vi "Update.vi"(8 "error in (no error)":errorcluster caption="entrée d'erreur (pas d'erreur)", 11 "Dual Fan en entrée":refnum<class "Dual Fan.lvclass">) -> (0 "error out":errorcluster caption="sortie d'erreur", 3 "Dual Fan en sortie":refnum<class "Dual Fan.lvclass">)   [LabVIEW 2015, in "Dual Fan.lvlib" / "Dual Fan.lvclass"]
uses:
  Dual Fan.lvclass
  Simulation/Simulation Data_Global.vi
  Simulation/Simulation.lvlib
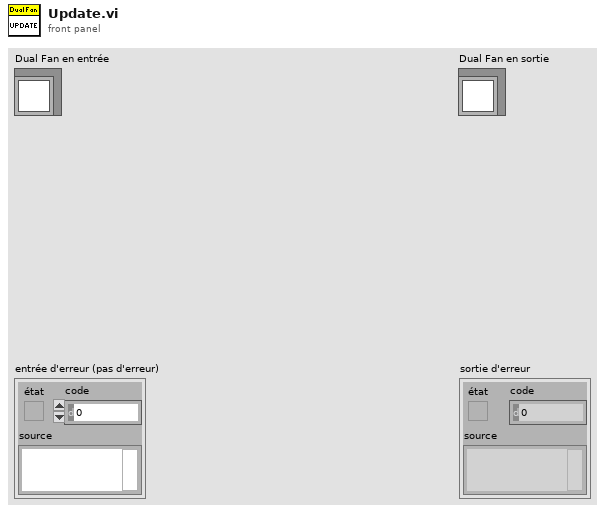
[diagram p1: front panel]
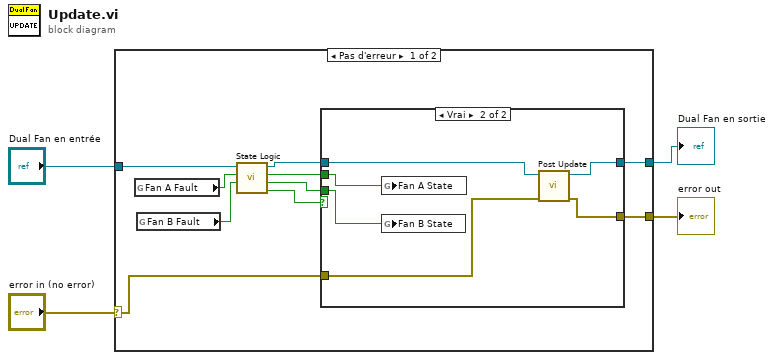
[diagram p0: block diagram]
diagram:
  n1 = case shown="Pas d'erreur" "error in (no error)" {
    selector: "error in (no error)" -> [w6 w23]
    tunnel: [w11 w24] -> w3
    tunnel: "Dual Fan en entrée" -> [w9 w24]
    tunnel: [w5 w23] -> w1
    frame No Error {
      n2 = global read "Simulation Data_Global.vi" "Fan A Fault"() -> (w8:bool)
      n3 = global read "Simulation Data_Global.vi" "Fan B Fault"() -> (w7:bool)
      n4 = call "State Logic.vi"("Fan B Fault"=w7, "Fan A Fault"=w8, "Dual Fan in"=w9) -> ("State Changed"=w14:bool, "Fan B State"=w13:bool, "Fan A State"=w12:bool, "Dual Fan out"=w10:refnum<class "Dual Fan.lvclass">)  [unwired: 5 in]
      n5 = case shown="Vrai" w14 {
        tunnel: w13 -> [_ w21]
        tunnel: w12 -> [_ w22]
        tunnel: [w16 w19] -> w11
        tunnel: w10 -> [w16 w20]
        tunnel: w6 -> [w15 w18]
        tunnel: [w15 w17] -> w5
        frame False {
        }
        frame True {
          n6 = global write "Simulation Data_Global.vi" "Fan A State"(w22) -> ()
          n7 = global write "Simulation Data_Global.vi" "Fan B State"(w21) -> ()
          n8 = call "Post Update.vi"("error in (no error)"=w18, "Dual Fan in"=w20) -> ("error out"=w17:errorcluster, "Dual Fan out"=w19:refnum<class "Dual Fan.lvclass">)  [unwired: 8 in]
        }
      }
    }
    frame Error {
    }
  }
  "error out" <- w1
  "Dual Fan en sortie" <- w3
